vi "Read RocketPlotHandle.vi"(8 "error in (no error)":errorcluster, 11 "SinglePlotPanel in":refnum<class "RocketPlotPanel.lvclass">) -> (0 "error out":errorcluster, 2 "RocketPlotHandle":refnum<class "RocketPlotHandle.lvclass">, 3 "SinglePlotPanel out":refnum<class "RocketPlotPanel.lvclass">)   [LabVIEW 2021, in "RocketPlot.lvlib" / "RocketPlotPanel.lvclass"]
uses:
  RocketPlotPanel.lvclass
  RocketPlotHandle/RocketPlotHandle.lvclass
  RocketPlotPanel.lvclass/RocketPlotPanel.ctl
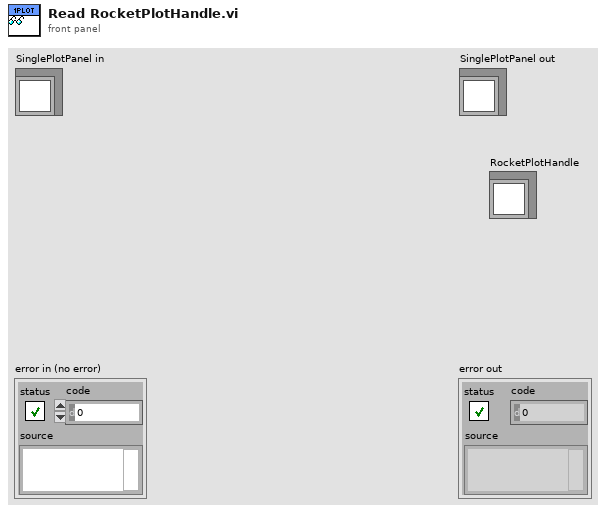
[diagram p1: front panel]
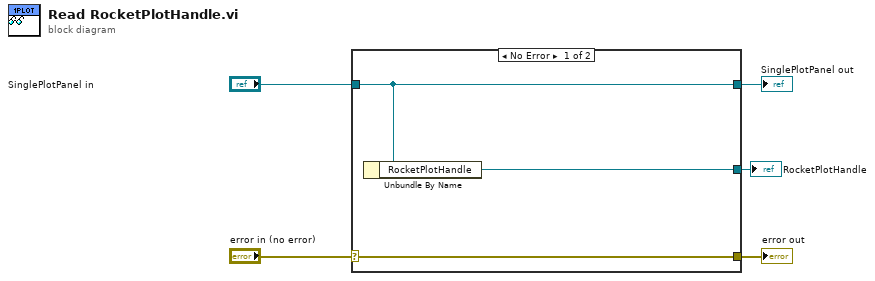
[diagram p0: block diagram]
diagram:
  n1 = case shown="No Error" "error in (no error)" {
    selector: "error in (no error)" -> [w8 w9]
    tunnel: [w8 w9] -> w4
    tunnel: [w7 w10] -> w2
    tunnel: "SinglePlotPanel in" -> [w7 w10]
    tunnel: [w6 _] -> w1
    frame No Error {
      n2 = Unbundle By Name(w7) -> ("RocketPlotHandle"=w6:refnum<class "RocketPlotHandle.lvclass">)
    }
    frame Error {
    }
  }
  "error out" <- w4
  "SinglePlotPanel out" <- w2
  "RocketPlotHandle" <- w1
